vi "GetHighestN1DFrom2D.vi"(1 "# Outputs":i32, 2 "Sort by Row #":i32, 3 "Array":dbl[][](array[numeric])) -> (0 "Out":dbl[][](array[numeric]))   [LabVIEW 2015]
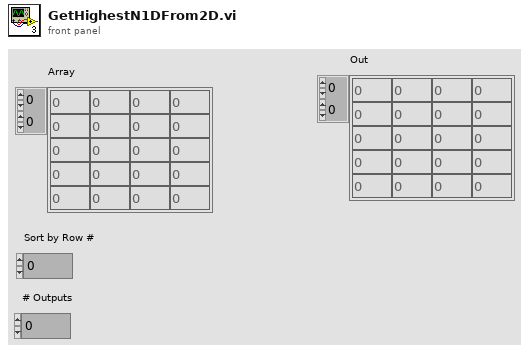
[diagram p1: front panel]
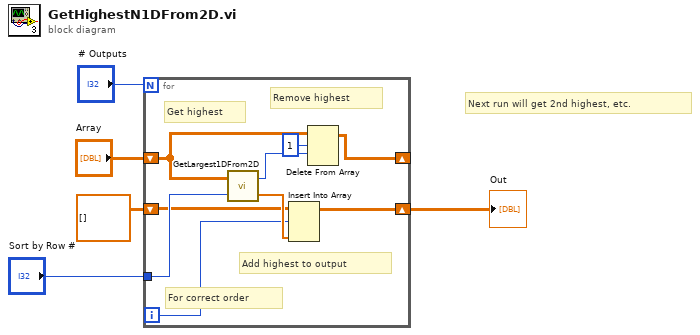
[diagram p0: block diagram]
diagram:
  # "Next run will get 2nd highest, etc."
  n1 = for {
    N: "# Outputs" -> [_]
    tunnel: "Sort by Row #" -> [w14]
    shift-right: [w11] -> w1
    shift-left: dbl[][] [] -> [w12]
    shift-right: [w7] -> _
    shift-left: "Array" -> [w10]
    i -> [w6]
    # "Add highest to output"
    # "Remove highest"
    # "Get highest"
    # "For correct order"
    n2 = call "GetLargest1DFrom2D.vi"("Row No."=w14, "2D Input"=w10) -> ("1D Output"=w13:dbl[], "max index(es)"=w9:i32)
    n3 = Insert Into Array(array=w12, index (row)=w6, new element=w13) -> (w11:dbl[][])  [unwired: 1 in]
    n4 = Delete From Array(array=w10, length=1, index (row)=w9) -> (array with subset deleted=w7:dbl[][])  [unwired: 1 in, 1 out]
  }
  "Out" <- w1
